vi "Write Experiment Parameter.vi"(10 "Experiment Parameters":T1, 11 "Data Analyser Reportin":refnum<class "Data Analyser Report.lvclass">) -> (3 "Data Analyser Report out":refnum<class "Data Analyser Report.lvclass">)   [LabVIEW 2013, in "Data Analyser Report.lvclass"]
uses:
  Data Analyser Report.lvclass
  Excel Interface/Excel Sheet/Write to Cell - String.vi
  Excel Interface/Excel Sheet/Write to Cell - Dbl.vi
  Excel Interface/Excel Sheet/Excel Sheet.lvclass
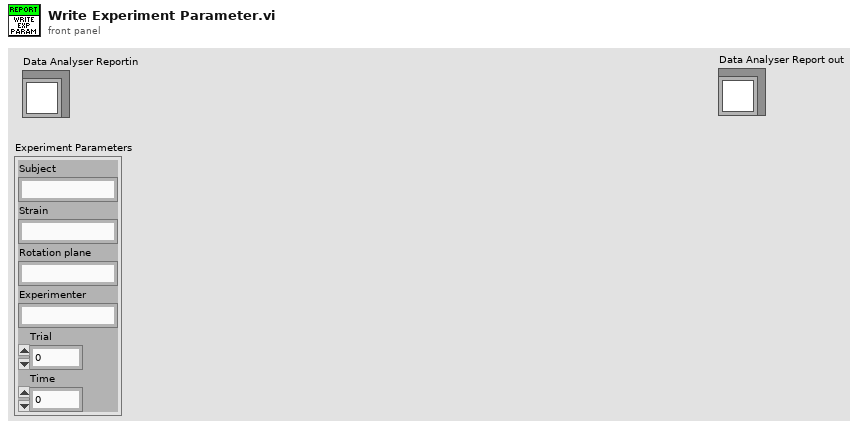
[diagram p1: front panel]
types:
  T1 = cluster{"Subject":string, "Strain":string, "Rotation plane":string, "Experimenter":string, "Trial":dbl, "Time":dbl}
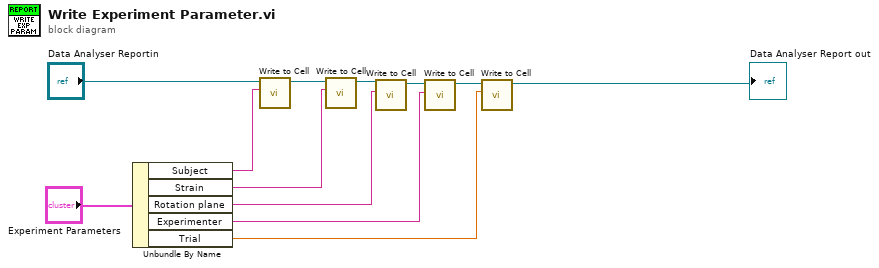
[diagram p0: block diagram]
diagram:
  n1 = Unbundle By Name("Experiment Parameters") -> ("Subject"=w10:string, "Strain"=w4:string, "Rotation plane"=w3:string, "Experimenter"=w2:string, "Trial"=w1:dbl)
  n2 = call-poly "Write to Cell.vi"("Value"=w10, "Excel Sheet in"="Data Analyser Reportin") -> ("Excel Sheet out"=w9:refnum<class "Data Analyser Report.lvclass">)  [unwired: 9 in]
  n3 = call-poly "Write to Cell.vi"("Value"=w4, "Excel Sheet in"=w9) -> ("Excel Sheet out"=w8:refnum<class "Data Analyser Report.lvclass">)  [unwired: 9 in]
  n4 = call-poly "Write to Cell.vi"("Value"=w3, "Excel Sheet in"=w8) -> ("Excel Sheet out"=w7:refnum<class "Data Analyser Report.lvclass">)  [unwired: 9 in]
  n5 = call-poly "Write to Cell.vi"("Value"=w2, "Excel Sheet in"=w7) -> ("Excel Sheet out"=w6:refnum<class "Data Analyser Report.lvclass">)  [unwired: 9 in]
  n6 = call-poly "Write to Cell.vi"("Value"=w1, "Excel Sheet in"=w6) -> ("Excel Sheet out"=→"Data Analyser Report out":refnum<class "Data Analyser Report.lvclass">)  [unwired: 9 in]
